vi "task_1.vi"() -> ()   [LabVIEW 2018]
panel:
  in  "stop":bool
  out "Meter":dbl(knob) scale=0.0..5.0
  out "data":dbl
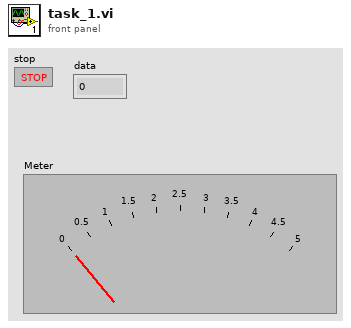
[diagram p1: front panel]
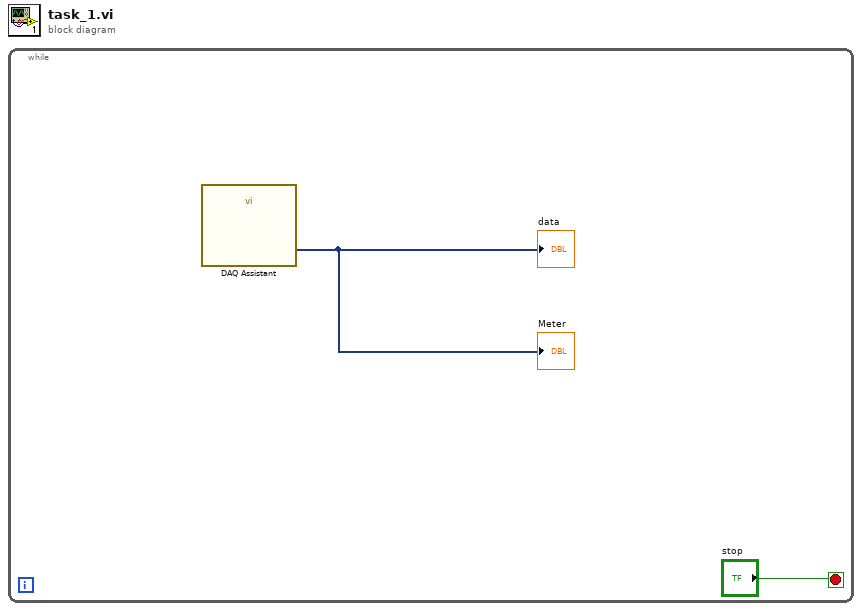
[diagram p0: block diagram]
diagram:
  n1 = while {
    stop <- "stop" stop-if-true
    n2 = call "DAQ Assistant"() -> ("data"=→"data" →"Meter":dynamicdata)  [unwired: 17 in, 2 out]
  }
